vi "4.5.vi"(0 "输入":dbl) -> (1 "随机数的值":i8, 2 "循环次数":i8)   [LabVIEW 2017]
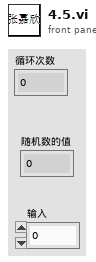
[diagram p1: front panel]
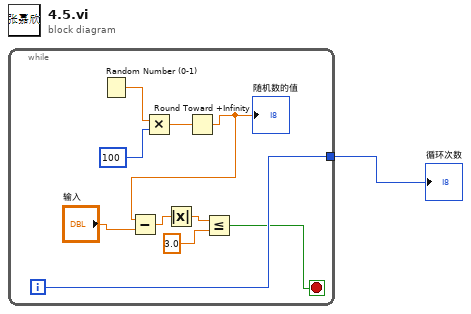
[diagram p0: block diagram]
diagram:
  n1 = while {
    tunnel: [w11] -> w1
    i -> [w11]
    stop <- w5 stop-if-true
    n2 = Random Number (0-1)() -> (number: 0 to 1=w10:dbl)
    n3 = Multiply(x=w10, y=100) -> (x*y=w8:dbl)
    n4 = Round Toward +Infinity(x=w8) -> (ceil(x): smallest int >= x=w4:dbl)
    "随机数的值" <- w4
    n5 = Subtract(x=w4, y="输入") -> (x-y=w3:dbl)
    n6 = Absolute Value(x=w3) -> (abs(x)=w2:dbl)
    n7 = Less Or Equal?(x=w2, y=3.0) -> (x <= y?=w5:bool)
  }
  "循环次数" <- w1
